vi "Butterfly_PullDown RCV.vi"(0 "Semiconductor Module Context":T2, 1 "RFPins":string[](array[string]), 2 "current level":dbl=0.01 format="%_6p", 3 "R Thresholds":dbl[](array[numeric]), 4 "Capacitance":bool=TRUE, 5 "error in (no error)":errorcluster, 6 "VNAs Measurement Parameters":T1, 7 "Start_v":dbl=10.0 format="%#_13g", 8 "C_TH_Delta":dbl=2.0, 9 "Stop_v":dbl=41.0 format="%#_13g", 11 "Step_v":dbl=1.0) -> (14 "Semiconductor Module Context Out":T2, 19 "error out":errorcluster)   [LabVIEW 2013]
uses:
  <vilib>/NI_TestStand_SemiconductorModule/NI_TestStand_Semiconductor_Module.lvlibp/PinMap/General/SemiconductorModuleContext.ctl
  VNA/VNAs Measurement Parameters.ctl
  <instrlib>/niDCPower/nidcpower.llb/niDCPower Wait For Event - Event.ctl
  <vilib>/NI_TestStand_SemiconductorModule/NI_TestStand_Semiconductor_Module.lvlibp/PinMap/DC Power/PinsToNIDCPowerSessions.vi
  <vilib>/NI_TestStand_SemiconductorModule/NI_TestStand_Semiconductor_Module.lvlibp/PinMap/General/Publish/PublishDataDoubleFunctionalTest.vi
  <vilib>/NI_TestStand_SemiconductorModule/NI_TestStand_Semiconductor_Module.lvlibp/PinMap/General/Publish/PublishDataDouble2D.vi
  <vilib>/NI_TestStand_SemiconductorModule/NI_TestStand_Semiconductor_Module.lvlibp
  VNA/Pin Map API/VNA Custom Instrument.lvlib
panel:
  in  "SMU_PD":refnum<k15>="4139_1"
  out "VPIs 2":dbl[](array[numeric])
  out "VRLs 2":dbl[](array[numeric])
  out "S0 steps":dbl[](array[numeric]) format="%#_3g"
  out "S1 steps":dbl[](array[numeric]) format="%#_3g"
  out "S2 steps":dbl[](array[numeric]) format="%#_3g"
  out "S3 steps":dbl[](array[numeric]) format="%#_3g"
  out "appended array":dbl[][](array[numeric]) format="%#_3g"
  out "VPIs":dbl[][](array[numeric]) format="%#_3g"
  out "VRLs":dbl[][](array[numeric]) format="%#_3g"
  out "C_Free":dbl[](array[numeric])
  out "Full R Array":dbl[][][](array[numeric])
  out "step":i32
  out "Instrument Session":refnum<k15>
  out "sites and pins loop iter":i32
  out "Channel List":string
  out "BF values":dbl[](array[numeric])
  out "BF Names":string[](array[string])
  out "R Array":dbl[](array[numeric])
  out "BFSamples":i32
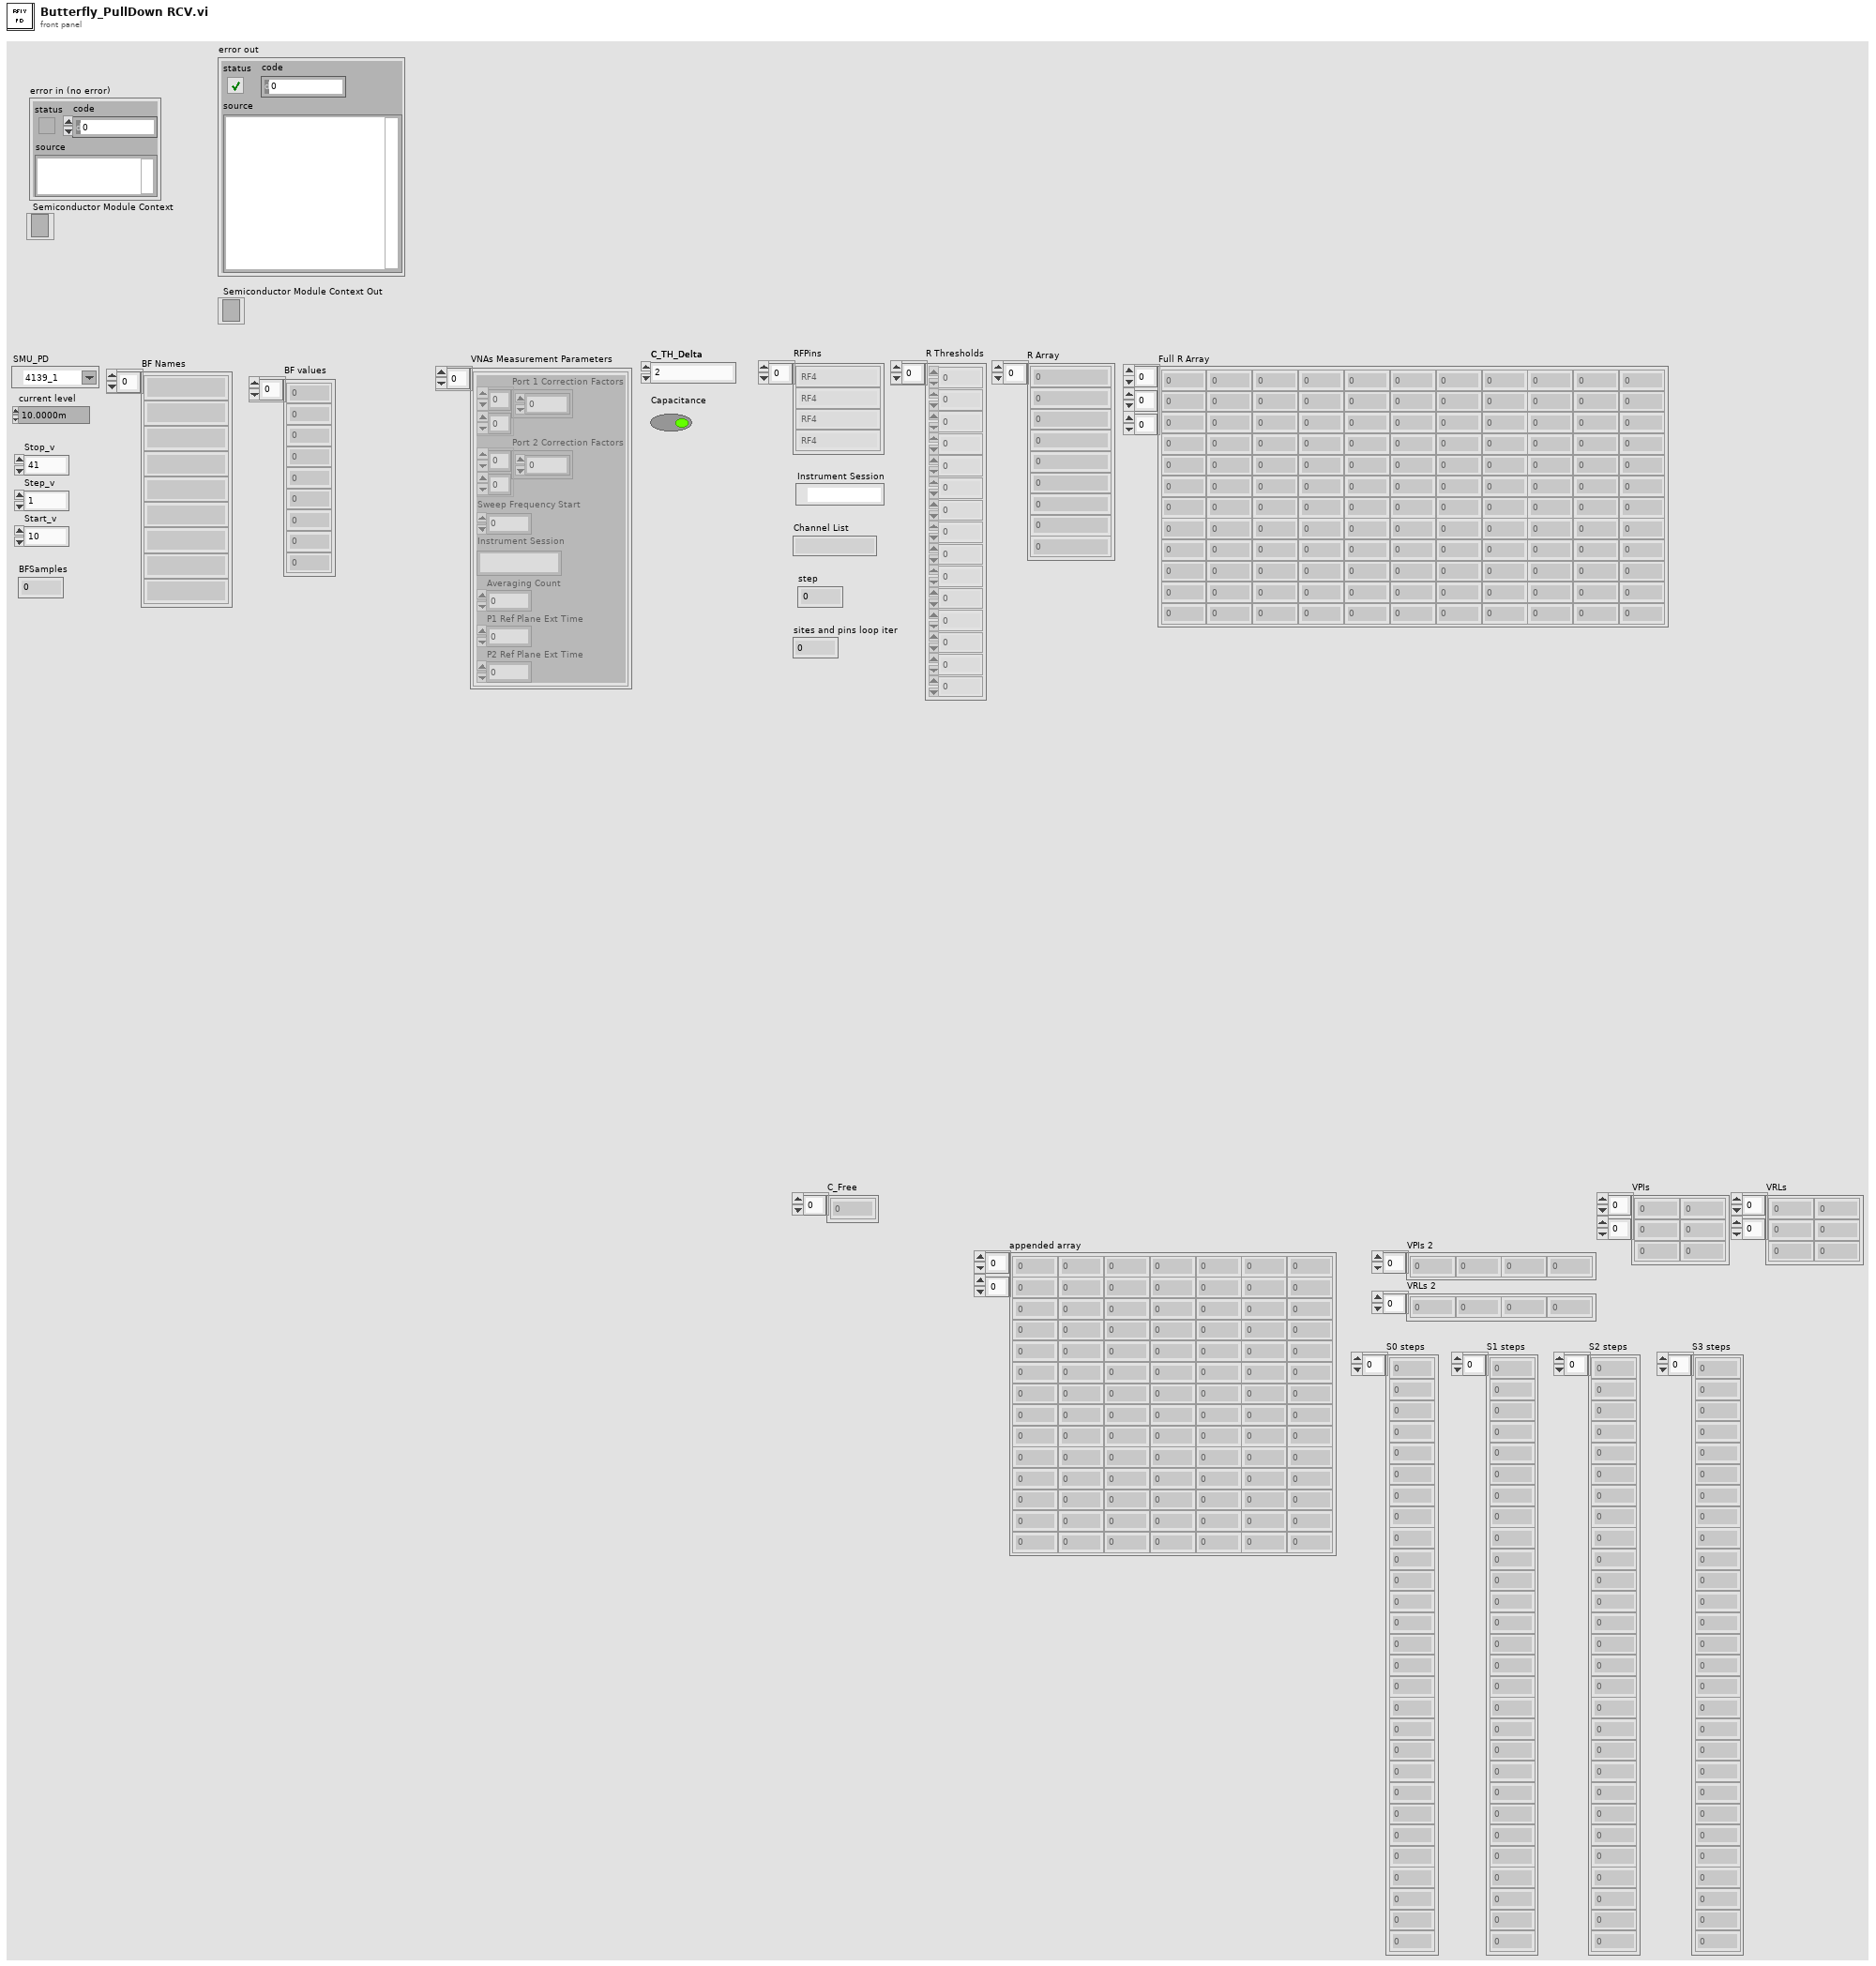
[diagram p1: front panel]
types:
  T1 = typedef "VNAs Measurement Parameters.ctl" = cluster{"Port 1 Correction Factors":cdb[][], "Port 2 Correction Factors":cdb[][], "Sweep Frequency Start":dbl, "Instrument Session":string, "Averaging Count":i32, "P1 Ref Plane Ext Time":dbl, "P2 Ref Plane Ext Time":dbl}[]
  T2 = typedef "NI_TestStand_Semiconductor_Module.lvlibp/SemiconductorModuleContext.ctl" = refnum<k7>
  T3 = typedef "niDCPower Wait For Event - Event.ctl" = i32
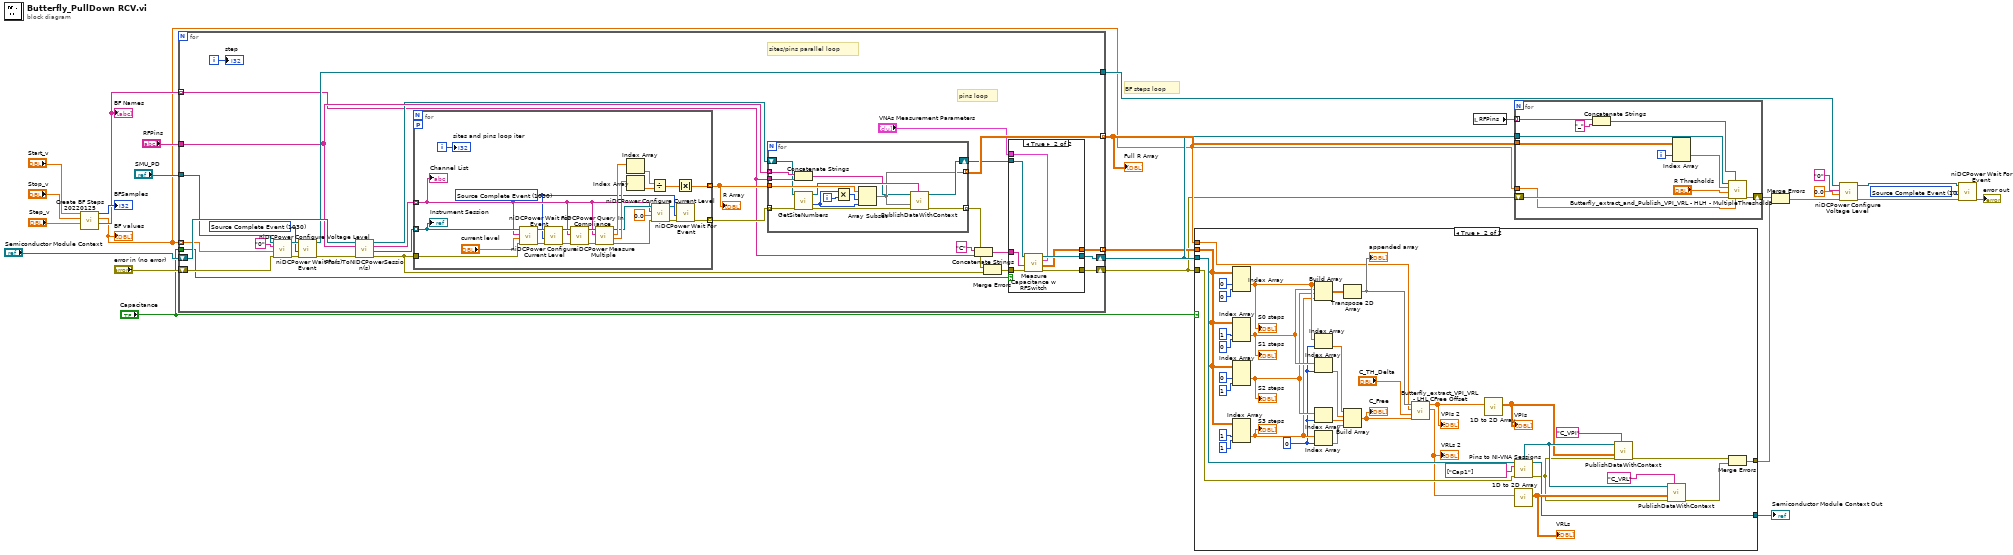
[diagram p0: block diagram]
diagram:
  w15 = T3 1030 items=["Source Complete Event"=1030, "Measure Complete Event"=1031, "Sequence Iteration Complete Event"=1032, "Sequence Engine Done Event"=1033, "Pulse Complete Event"=1051, "Ready For Pulse Trigger Event"=1052] ("event")
  # "BF steps loop"
  n1 = call "Create BF Steps 20220125.vi"("Step_v"="Step_v", "Stop_v"="Stop_v", "Start_v"="Start_v") -> ("BF Names"=w13:string[], "BF values"=w7:dbl[], "BFSamples"=→"BFSamples":i32)  [unwired: 6 in]
  "BF Names" <- w13
  "BF values" <- w7
  n2 = for {
    shift-right: [w34] -> w6
    shift-left: "error in (no error)" -> [w53]
    tunnel: w7 -> [w51] mode=indexing
    tunnel: "SMU_PD" -> [w50]
    tunnel: [w49] -> w19
    shift-right: [w29] -> w9
    shift-left: "Semiconductor Module Context" -> [w57]
    tunnel: "RFPins" -> [w43]
    tunnel: w13 -> [w32] mode=indexing
    tunnel: [w40] -> w11 mode=indexing
    tunnel: "Capacitance" -> [w30]
    tunnel: [w28] -> w8 mode=indexing
    i -> [w45]
    w55 = T3 1030 items=["Source Complete Event"=1030, "Measure Complete Event"=1031, "Sequence Iteration Complete Event"=1032, "Sequence Engine Done Event"=1033, "Pulse Complete Event"=1051, "Ready For Pulse Trigger Event"=1052] ("event")
    # "pins loop"
    # "sites/pins parallel loop"
    n3 = call <instrlib>:"niDCPower Configure Voltage Level.vi"("error in (no error)"=w53, "voltage level"=w51, "channel name"="0", "instrument handle"=w50) -> ("error out"=w54:errorcluster, "instrument handle out"=w56:refnum<k15>)  [unwired: 6 in]
    n4 = call <instrlib>:"niDCPower Wait For Event.vi"("error in (no error)"=w54, "event"=w55, "instrument handle"=w56) -> ("error out"=w52:errorcluster, "instrument handle out"=w49:refnum<k15>)  [unwired: 7 in]
    n5 = call-poly <vilib>:"Pin(s)ToNIDCPowerSession(s).vi"("error in (no error)"=w52, "Pins"=w43, "Semiconductor Module Context"=w57) -> ("error out"=w47:errorcluster, "Instrument Sessions"=w48:refnum<k15>[], "Channel Lists"=w46:string[], "Semiconductor Module Context Out"=w41:T2)  [unwired: 4 in, 1 out]
    n6 = for {
      tunnel: w46 -> [w85] mode=indexing
      tunnel: w48 -> [w90] mode=indexing
      tunnel: w47 -> [w91]
      tunnel: [w92] -> w42 mode=indexing
      tunnel: [w86] -> w38 mode=indexing
      workers-P: _ -> [_]
      i -> [w89]
      w84 = T3 1030 items=["Source Complete Event"=1030, "Measure Complete Event"=1031, "Sequence Iteration Complete Event"=1032, "Sequence Engine Done Event"=1033, "Pulse Complete Event"=1051, "Ready For Pulse Trigger Event"=1052] ("event")
      n7 = call <instrlib>:"niDCPower Configure Current Level.vi"("error in (no error)"=w91, "current level"="current level", "channel name"=w85, "instrument handle"=w90) -> ("error out"=w100:errorcluster, "instrument handle out"=w99:refnum<k15>)  [unwired: 6 in]
      n8 = call <instrlib>:"niDCPower Wait For Event.vi"("error in (no error)"=w100, "event"=w84, "instrument handle"=w99) -> ("error out"=w104:errorcluster, "instrument handle out"=w103:refnum<k15>)  [unwired: 7 in]
      n9 = call <instrlib>:"niDCPower Query In Compliance.vi"("error in (no error)"=w104, "channel name"=w85, "instrument handle"=w103) -> ("error out"=w101:errorcluster, "instrument handle out"=w102:refnum<k15>)  [unwired: 6 in, 1 out]
      n10 = call <instrlib>:"niDCPower Measure Multiple.vi"("error in (no error)"=w101, "channel name"=w85, "instrument handle"=w102) -> ("error out"=w88:errorcluster, "current measurements"=w93:dbl[], "voltage measurements"=w94:dbl[], "instrument handle out"=w87:refnum<k15>)  [unwired: 5 in]
      n11 = Index Array(array=w94) -> (element=w96:dbl)  [unwired: 1 in]
      n12 = Index Array(array=w93) -> (element=w95:dbl)  [unwired: 1 in]
      n13 = Divide(x=w96, y=w95) -> (x/y=w97:dbl)
      n14 = call <instrlib>:"niDCPower Configure Current Level.vi"("error in (no error)"=w88, "current level"=0.0, "channel name"=w85, "instrument handle"=w87) -> ("error out"=w83:errorcluster, "instrument handle out"=w82:refnum<k15>)  [unwired: 6 in]
      n15 = Absolute Value(x=w97) -> (abs(x)=w92:dbl)
      n16 = call <instrlib>:"niDCPower Wait For Event.vi"("error in (no error)"=w83, "event"=w84, "instrument handle"=w82) -> ("error out"=w86:errorcluster)  [unwired: 7 in, 1 out]
      "Channel List" <- w85
      "sites and pins loop iter" <- w89
      "Instrument Session" <- w90
    }
    "R Array" <- w42
    n17 = for {
      tunnel: [w75] -> w44 mode=indexing
      tunnel: w43 -> [w79] mode=indexing
      tunnel: w42 -> [w76]
      tunnel: w32 -> [w78]
      shift-right: [w73] -> w37
      shift-left: w41 -> [w70]
      tunnel: [w72] -> w40 mode=indexing
      tunnel: w38 -> [w67] mode=indexing
      i -> [w80]
      n18 = Concatenate Strings(w79, w78) -> (w74:string)
      n19 = call <vilib>:"GetSiteNumbers.vi"("error in (no error)"=w67, "Semiconductor Module Context"=w70) -> ("error out"=w71:errorcluster, "Number Of Sites"=w68:i32, "Semiconductor Module Context Out"=w69:T2)  [unwired: 6 in, 1 out]
      n20 = Multiply(x=w68, y=w80) -> (x*y=w77:i32)
      n21 = Array Subset(array=w76, index=w77, length=w68) -> (w72:dbl[])
      n22 = call-poly <vilib>:"PublishDataWithContext.vi"("Published Data Id"=w74, "error in (no error)"=w71, "Data In"=w72, "Semiconductor Module Context"=w69) -> ("error out"=w75:errorcluster, "Semiconductor Module Context Out"=w73:T2)  [unwired: 6 in]
    }
    n23 = Concatenate Strings("C" ("string"), w32) -> (w31:string)
    n24 = Merge Errors(w44, w47) -> (w35:errorcluster)
    n25 = case shown="True" w30 {
      tunnel: w37 -> [w59 w66]
      tunnel: [w59 w65] -> w29
      tunnel: [w58 w64] -> w34
      tunnel: w31 -> [_ w63]
      tunnel: "VNAs Measurement Parameters" -> [_ w62]
      tunnel: [_ w60] -> w28
      tunnel: w35 -> [w58 w61]
      frame False {
      }
      frame True {
        n26 = call "Measure Capacitance w RFSwitch.vi"("VNAs Measurement Parameters"=w62, "error in (no error)"=w61, "Measurement Id"=w63, "Semiconductor Module Context"=w66) -> ("error out"=w64:errorcluster, "Multisite Cap Data"=w60:dbl[][], "Semiconductor Module Context Out"=w65:T2)  [unwired: 5 in]
      }
    }
    "step" <- w45
  }
  "Full R Array" <- w11
  n27 = case shown="True" "Capacitance" {
    tunnel: [w105 w125] -> w1
    tunnel: [w106 w143] -> w3
    tunnel: w9 -> [w105 w142]
    tunnel: w6 -> [w106 w138]
    tunnel: w7 -> [_ w110]
    tunnel: w8 -> [_ w129]
    frame False {
    }
    frame True {
      w118 = 0 ("index")
      n28 = Index Array(array=w129, index (dim 1)=0 ("disabled index (row)"), index (dim 2)=0 ("disabled index (col)")) -> (element=w122:dbl[])  [unwired: 1 in]
      "S0 steps" <- w122
      n29 = Index Array(array=w129, index (dim 1)=1 ("index (row)"), index (dim 2)=0 ("index (col)")) -> (element=w121:dbl[])  [unwired: 1 in]
      "S1 steps" <- w121
      n30 = Index Array(array=w129, index (dim 1)=0 ("index (row)"), index (dim 2)=1 ("index (col)")) -> (element=w120:dbl[])  [unwired: 1 in]
      "S2 steps" <- w120
      n31 = Index Array(array=w129, index (dim 1)=1 ("index (row)"), index (dim 2)=1 ("index (col)")) -> (element=w119:dbl[])  [unwired: 1 in]
      "S3 steps" <- w119
      n32 = Build Array(w122, w121, w120, w119) -> (w113:dbl[][])
      n33 = Index Array(array=w122, index=w118) -> (element=w117:dbl)
      n34 = Index Array(array=w121, index=w118) -> (element=w116:dbl)
      n35 = Index Array(array=w120, index=w118) -> (element=w115:dbl)
      n36 = Index Array(array=w119, index=w118) -> (element=w114:dbl)
      n37 = Transpose 2D Array(2D array=w113) -> (transposed array=w111:dbl[][])
      "appended array" <- w111
      n38 = Build Array(w117, w116, w115, w114) -> (w112:dbl[])
      "C_Free" <- w112
      n39 = call "Butterfly_extract_VPI_VRL - LHL CFree Offset.vi"("C_Free"=w112, "Delta"="C_TH_Delta", "Voltage Array"=w110, "Result Array In"=w111) -> ("VRLs"=w107:dbl[], "VPIs"=w108:dbl[])  [unwired: 6 in]
      "VPIs 2" <- w108
      "VRLs 2" <- w107
      n40 = call "1D to 2D Array.vi"("1D Array"=w108) -> ("2D Array"=w127:dbl[][])  [unwired: 10 in]
      "VPIs" <- w127
      n41 = call "Pins to NI-VNA Sessions.vi"("Semiconductor Module Context"=w142, "Pins"=string[] ["Cap1"] ("Capacitance Pins"), "error in (no error)"=w138) -> ("Pin Query Context"=w128:refnum<class "MultiplePinMultipleSessionQueryContext.lvclass">, "Semiconductor Module Context Out"=w125:T2, "error out"=w123:errorcluster)  [unwired: 8 in, 2 out]
      n42 = call "1D to 2D Array.vi"("1D Array"=w107) -> ("2D Array"=w141:dbl[][])  [unwired: 10 in]
      "VRLs" <- w141
      n43 = call-poly <vilib>:"PublishDataWithContext.vi"("Published Data Id"="C_VPI", "error in (no error)"=w123, "Data In"=w127, "Pin Query Context"=w128) -> ("error out"=w124:errorcluster)  [unwired: 6 in, 1 out]
      n44 = call-poly <vilib>:"PublishDataWithContext.vi"("Published Data Id"="C_VRL", "error in (no error)"=w123, "Data In"=w141, "Pin Query Context"=w128) -> ("error out"=w144:errorcluster)  [unwired: 6 in, 1 out]
      n45 = Merge Errors(w124, w144) -> (w143:errorcluster)
    }
  }
  "Semiconductor Module Context Out" <- w1
  n46 = local read "RFPins"() -> (w12:string[])
  n47 = for {
    tunnel: w12 -> [w149] mode=indexing
    tunnel: w11 -> [w154]
    shift-right: [w150] -> w4
    shift-left: w6 -> [w151]
    tunnel: w9 -> [w146]
    tunnel: w7 -> [w145]
    i -> [w155]
    n48 = Concatenate Strings(w149, "_" ("string")) -> (w147:string)
    n49 = Index Array(array=w154, index (dim 1)=w155) -> (element=w152:dbl[][])  [unwired: 2 in]
    n50 = call "Butterfly_extract_and_Publish_VPI_VRL - HLH - MultipleThresholds.vi"("Voltages Array"=w145, "ID Prefix"=w147, "error in (no error)"=w151, "Thresholds"="R Thresholds", "Result Array In"=w152, "Semiconductor Module Context"=w146) -> ("error out"=w150:errorcluster)  [unwired: 5 in]
  }
  n51 = Merge Errors(w4, w3) -> (w2:errorcluster)
  n52 = call <instrlib>:"niDCPower Configure Voltage Level.vi"("error in (no error)"=w2, "voltage level"=0.0, "channel name"="0", "instrument handle"=w19) -> ("error out"=w18:errorcluster, "instrument handle out"=w16:refnum<k15>)  [unwired: 6 in]
  n53 = call <instrlib>:"niDCPower Wait For Event.vi"("error in (no error)"=w18, "event"=w15, "instrument handle"=w16) -> ("error out"=→"error out":errorcluster)  [unwired: 7 in, 1 out]
